vi "Induction Matrix Model.vi"(11 "Build Specifications":T1={"Length (m)"=3, "Width (m)"=3, "Height (m)"=4, "Matrix Blocks"={"Basic Cells"=0, "Advanced Cells"=0, "Elite Cells"=0, "Ultimate Cells"=0, "Basic Providers"=0, "Advanced Providers"=0, "Elite Providers"=0, "Ultimate Providers"=0}} {"Height (m)" min=3 max=18 step=1; "Width (m)" min=3 max=18 step=1; "Length (m)" min=3 max=18 step=1}) -> (0 "Provider Rate (kFE/t)":ext, 1 "Storage (GFE)":ext, 2 "Fits In Structure?":bool, 3 "Total Blocks":u64, 4 "Induction Matrix Build Properties":T2)   [LabVIEW 2026]
uses:
  Induction Matrix Build Properties.ctl
  Induction Matrix Build Specifications.ctl
  45dc50cf-dc3e-764d-baf4-482615fca8eb.vi
  a49f6723-8312-4e4d-8470-a6d78d25dee5.vi
panel:
  # "Induction Matrix Info"
  # "8GJ\n64GJ\n512GJ\n4TJ"
  # "256kJ\n2.048MJ\n16.384MJ\n131.072MJ"
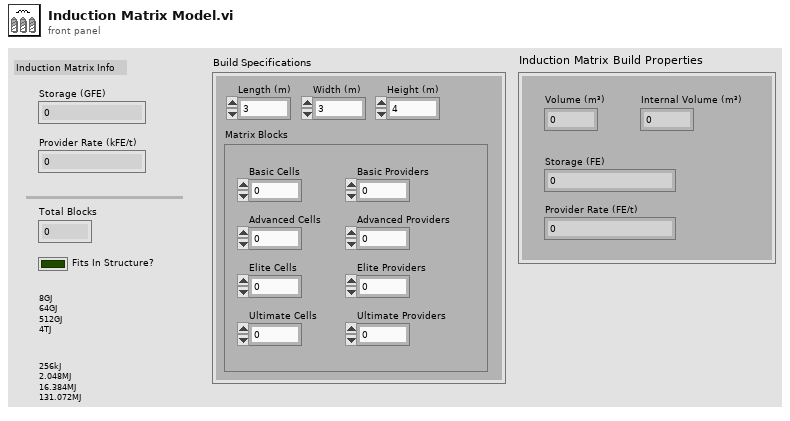
[diagram p1: front panel]
types:
  T1 = typedef "Induction Matrix Build Specifications.ctl" = cluster{"Length (m)":i32, "Width (m)":i32, "Height (m)":i32, "Matrix Blocks":cluster{"Basic Cells":u64, "Advanced Cells":u64, "Elite Cells":u64, "Ultimate Cells":u64, "Basic Providers":u64, "Advanced Providers":u64, "Elite Providers":u64, "Ultimate Providers":u64}}
  T2 = typedef "Induction Matrix Build Properties.ctl" = cluster{"Internal Volume (m³)":i32, "Volume (m³)":i32, "Storage (FE)":ext, "Provider Rate (FE/t)":ext}
  T3 = cluster{"Basic Cells":u64, "Advanced Cells":u64, "Elite Cells":u64, "Ultimate Cells":u64, "Basic Providers":u64, "Advanced Providers":u64, "Elite Providers":u64, "Ultimate Providers":u64}
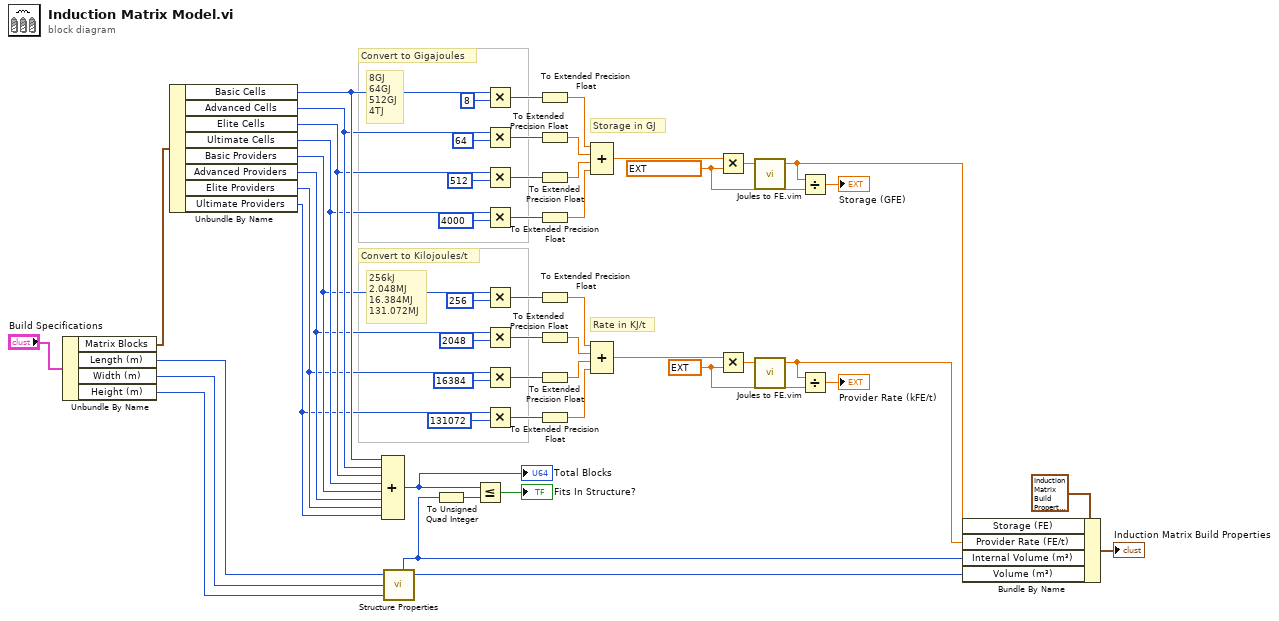
[diagram p0: block diagram]
diagram:
  w33 = ext 1000000000.0 ("y")
  w34 = ext 1000.0 ("y")
  # "Rate in KJ/t"
  # "Storage in GJ"
  # "Convert to Kilojoules/t"
  # "256kJ\n2.048MJ\n16.384MJ\n131.072MJ"
  # "8GJ\n64GJ\n512GJ\n4TJ"
  # "Convert to Gigajoules"
  n1 = Unbundle By Name("Build Specifications") -> ("Matrix Blocks"=w4:T3, "Length (m)"=w3:i32, "Width (m)"=w1:i32, "Height (m)"=w2:i32)
  n2 = Unbundle By Name(w4) -> ("Basic Cells"=w21:u64, "Advanced Cells"=w20:u64, "Elite Cells"=w19:u64, "Ultimate Cells"=w18:u64, "Basic Providers"=w17:u64, "Advanced Providers"=w16:u64, "Elite Providers"=w15:u64, "Ultimate Providers"=w14:u64)
  n3 = Compound Arithmetic op=ADD(w21, w20, w19, w18, w17, w16, w15, w14) -> (w45:u64)
  "Total Blocks" <- w45
  n4 = call "Structure Properties.vi"("Length"=w3, "Width"=w1, "Height"=w2) -> ("Inner Volume"=w7:i32, "Volume"=w6:i32)  [unwired: 2 in, 3 out]
  n5 = To Unsigned Quad Integer(1:w7) -> (0:w22:u64)
  n6 = Less Or Equal?(x=w45, y=w22) -> (x <= y?=→"Fits In Structure?":bool)
  n7 = Multiply(x=w21, y=u64 8) -> (x*y=w44:u64)
  n8 = Multiply(x=w20, y=u64 64) -> (x*y=w43:u64)
  n9 = Multiply(x=w19, y=u64 512) -> (x*y=w41:u64)
  n10 = Multiply(x=w18, y=u64 4000) -> (x*y=w42:u64)
  n11 = Multiply(x=w17, y=u64 256) -> (x*y=w40:u64)
  n12 = Multiply(x=w16, y=u64 2048) -> (x*y=w39:u64)
  n13 = Multiply(x=w15, y=u64 16384) -> (x*y=w38:u64)
  n14 = Multiply(x=w14, y=u64 131072) -> (x*y=w37:u64)
  n15 = To Extended Precision Float(1:w44) -> (0:w32:ext)
  n16 = To Extended Precision Float(1:w43) -> (0:w31:ext)
  n17 = To Extended Precision Float(1:w41) -> (0:w30:ext)
  n18 = To Extended Precision Float(1:w42) -> (0:w29:ext)
  n19 = To Extended Precision Float(1:w40) -> (0:w28:ext)
  n20 = To Extended Precision Float(1:w39) -> (0:w27:ext)
  n21 = To Extended Precision Float(1:w38) -> (0:w26:ext)
  n22 = To Extended Precision Float(1:w37) -> (0:w25:ext)
  n23 = Compound Arithmetic op=ADD(w32, w31, w30, w29) -> (w35:ext)
  n24 = Compound Arithmetic op=ADD(w28, w27, w26, w25) -> (w36:ext)
  n25 = Multiply(x=w35, y=w33) -> (x*y=w24:ext)
  n26 = Multiply(x=w36, y=w34) -> (x*y=w23:ext)
  n27 = call "Joules to FE.vim"("J"=w24) -> ("FE"=w9:ext)  [unwired: 4 in]
  n28 = call "Joules to FE.vim"("J"=w23) -> ("FE"=w8:ext)  [unwired: 4 in]
  n29 = Divide(x=w9, y=w33) -> (x/y=→"Storage (GFE)":ext)
  n30 = Divide(x=w8, y=w34) -> (x/y=→"Provider Rate (kFE/t)":ext)
  n31 = Bundle By Name(cluster=T2 {"Internal Volume (m³)"=0, "Volume (m³)"=0, "Storage (FE)"=0.0, "Provider Rate (FE/t)"=0.0} ("Induction Matrix Build Properties"), "Storage (FE)"=w9, "Provider Rate (FE/t)"=w8, "Internal Volume (m³)"=w7, "Volume (m³)"=w6) -> (→"Induction Matrix Build Properties":T2)
